vi "读取输入控件值ini.vi"(8 "错误输入（无错误）":errorcluster, 10 "appended path":path, 11 "VI输入":refnum<vi>) -> (0 "错误输出":errorcluster)   [LabVIEW 2016]
uses:
  <vilib>/Utility/config.llb/NI_LVConfig.lvlib
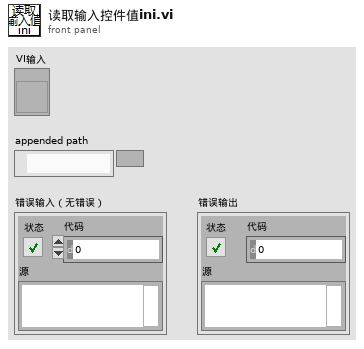
[diagram p1: front panel]
types:
  T1 = typedef "NI_LVConfig.lvlib/Config Data RefNum.ctl" = refnum<k1>
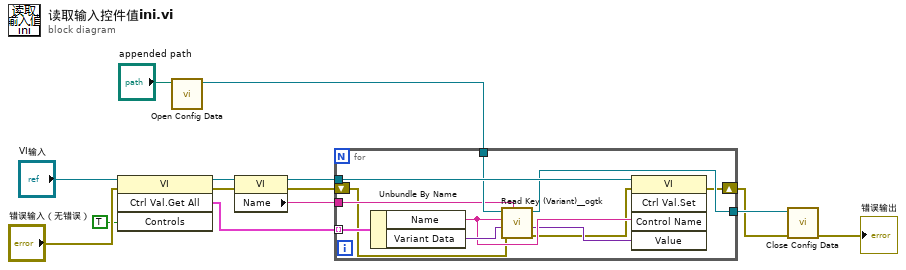
[diagram p0: block diagram]
diagram:
  n1 = invoke class="VI" method="Ctrl Val.Get All"(reference="VI输入", error in="错误输入（无错误）", "Controls"=TRUE ("控件")) -> (reference out=w14:refnum<vi>, error out=w13:errorcluster, "Get All Control Values Variant"=w8:cluster{"Name":string, "Variant Data":variant}[])  [unwired: 1 in, 1 out]
  n2 = call <vilib>:"Open Config Data.vi"("configuration file path"="appended path") -> ("refnum"=w10:T1)  [unwired: 8 in, 2 out]
  n3 = property class="VI"(reference=w14, error in=w13) -> (reference out=w9:refnum<vi>, error out=w4:errorcluster, "Name"=w7:string)
  n4 = for {
    tunnel: w9 -> [w25]
    tunnel: w10 -> [w24]
    tunnel: w8 -> [w23] mode=indexing
    tunnel: w7 -> [w22]
    tunnel: [w18] -> w6
    shift-right: [w15] -> w3
    shift-left: w4 -> [w17]
    n5 = Unbundle By Name(w23) -> ("Name"=w20:string, "Variant Data"=w21:variant)
    n6 = call <userlib>:"Read Key (Variant)__ogtk.vi"("section"=w22, "error in (no error)"=w17, "type"=w21, "key (optional)"=w20, "refnum"=w24) -> ("error out"=w16:errorcluster, "key-value"=w19:variant, "refnum out"=w18:T1)  [unwired: 3 in, 1 out]
    n7 = invoke class="VI" method="Ctrl Val.Set"(reference=w25, error in=w16, "Control Name"=w20, "Value"=w19) -> (error out=w15:errorcluster)  [unwired: 1 in, 4 out]
  }
  n8 = call <vilib>:"Close Config Data.vi"("error in (no error)"=w3, "refnum"=w6) -> ("error out"=→"错误输出":errorcluster)  [unwired: 8 in, 1 out]
